vi "VISAGlobal.vi"() -> ()   [LabVIEW 2023]
panel:
  in  "VISA":refnum<visa-resource-name>
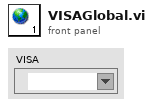
[diagram p1: front panel]
diagram:
